vi "Norm_array.vi"(11 "Array":dbl[](array[numeric])) -> (3 "Normed Array":dbl[](array[numeric]))   [LabVIEW 2018]
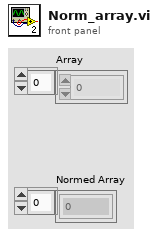
[diagram p1: front panel]
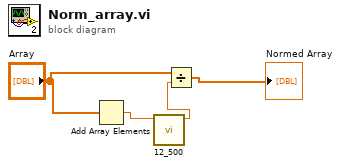
[diagram p0: block diagram]
diagram:
  n1 = Add Array Elements(numeric array="Array") -> (sum=w2:dbl)
  n2 = call "12_500.vi"("Numeric in"=w2) -> ("Numeric out"=w1:dbl)  [unwired: 10 in]
  n3 = Divide(x="Array", y=w1) -> (x/y=→"Normed Array":dbl[])
